vi "Add Connection to List (data structure)vi.vi"(8 "error in (no error)":errorcluster, 10 "Connection":T1, 11 "connection list":T1[](array[typedef])) -> (0 "error out":errorcluster, 1 "added":bool, 3 "connection list":T1[](array[typedef]))   [LabVIEW 2017, in "Switch Scripting.lvlib"]
uses:
  Switch Scripting.lvlib
  Connection.ctl
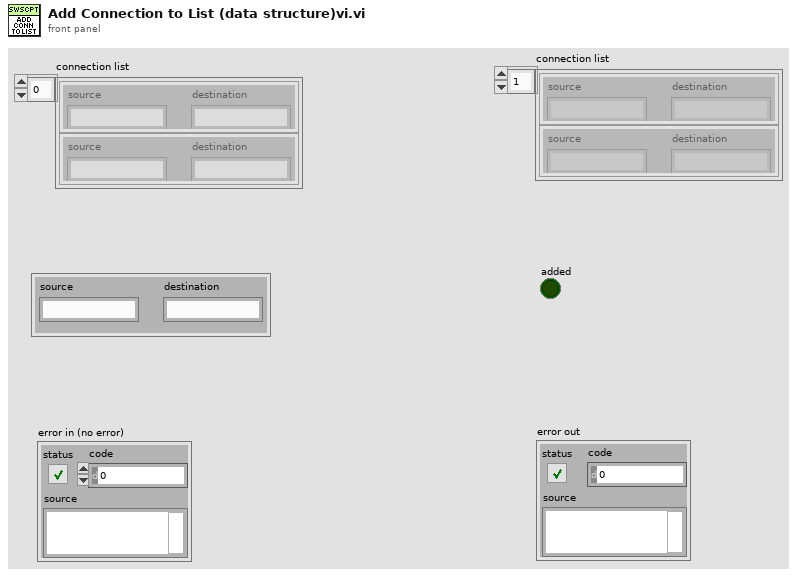
[diagram p1: front panel]
types:
  T1 = typedef "Switch Scripting.lvlib/Connection.ctl" = cluster{"source":string, "destination":string}
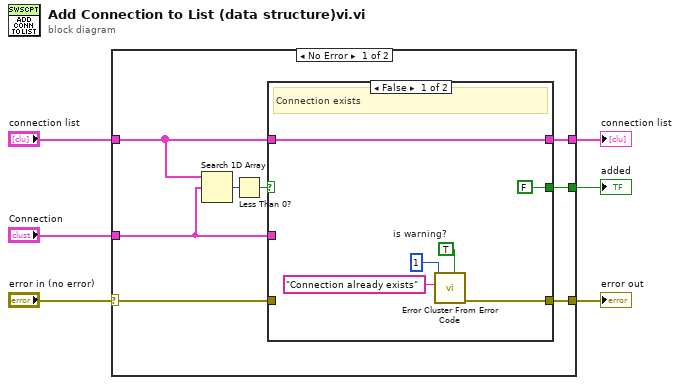
[diagram p0: block diagram]
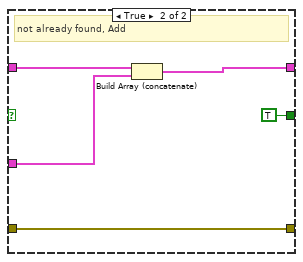
[diagram p2: hidden frame]
diagram:
  n1 = case shown="No Error" "error in (no error)" {
    selector: "error in (no error)" -> [w14 w27]
    tunnel: [w13 w27] -> w6
    tunnel: [w7 w26] -> w5
    tunnel: "connection list" -> [w8 w26]
    tunnel: "Connection" -> [w9 _]
    tunnel: [w10 _] -> w1
    frame No Error {
      n2 = Search 1D Array(1D array=w8, element=w9) -> (index of element=w12:i32)  [unwired: 1 in]
      n3 = Less Than 0?(x=w12) -> (x < 0?=w11:bool)
      n4 = case shown="False" w11 {
        tunnel: w14 -> [_ w25]
        tunnel: [w18 w25] -> w13
        tunnel: [FALSE TRUE] -> w10
        tunnel: w8 -> [w15 w23]
        tunnel: w9 -> [_ w22]
        tunnel: [w15 w21] -> w7
        frame False {
          w19 = TRUE  # is warning?
          # "Connection exists"
          n5 = call <vilib>:"Error Cluster From Error Code.vi"("is warning? (False)"=w19, "error message (\"\")"="Connection already exists" ("error message (\"\")"), "error code (0)"=1) -> ("error out"=w18:errorcluster)  [unwired: 6 in]
        }
        frame True {
          # "not already found, Add"
          n6 = Build Array (concatenate)(w23, w22) -> (w21:T1[])
        }
      }
    }
    frame Error {
    }
  }
  "error out" <- w6
  "connection list" <- w5
  "added" <- w1
